vi "Sort Classes by Name.vi"(8 "error in (no error)":errorcluster, 11 "Classes":refnum<vi>[](array[refnum])) -> (0 "error out":errorcluster, 3 "Sorted Classes":refnum<vi>[](array[refnum]))   [LabVIEW 2020, in "Peek Window.lvlib" / "Dynamic Dispatch VI Type.lvclass"]
uses:
  Dynamic Dispatch VI Type.lvclass
  Dynamic Dispatch VI Type.lvclass/Dynamic Dispatch VI Type.ctl
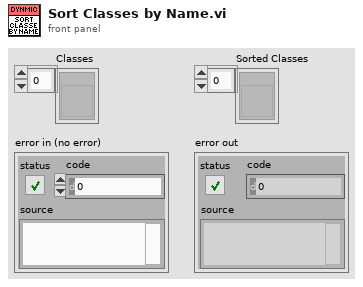
[diagram p1: front panel]
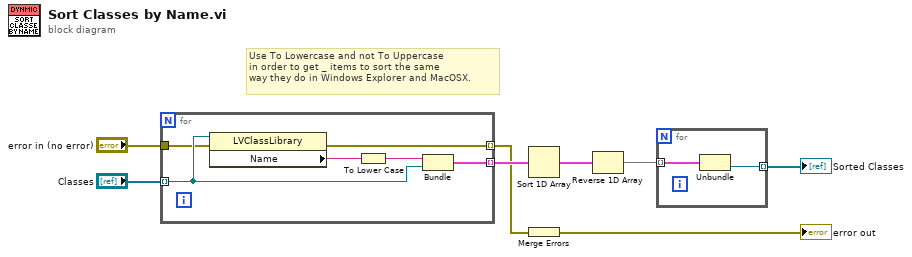
[diagram p0: block diagram]
diagram:
  # "Use To Lowercase and not To Uppercase\nin order to get _ items to sort the same\nway they do in Windows Explorer and MacOSX."
  n1 = for {
    tunnel: "Classes" -> [w13] mode=indexing
    tunnel: [w12] -> w4 mode=indexing
    tunnel: "error in (no error)" -> [w10]
    tunnel: [w9] -> w2 mode=indexing
    n2 = property class="LVClassLibrary"(reference=w13, error in=w10) -> (error out=w9:errorcluster, "Name"=w14:string)  [unwired: 1 out]
    n3 = To Lower Case(string=w14) -> (all lower case string=w11:string)
    n4 = Bundle(w11, w13) -> (w12:cluster{string, refnum<vi>})  [unwired: 1 in]
  }
  n5 = Sort 1D Array(array=w4) -> (sorted array=w5:cluster{string, refnum<vi>}[])
  n6 = Merge Errors(w2) -> (→"error out":errorcluster)
  n7 = Reverse 1D Array(array=w5) -> (reversed array=w8:cluster{string, refnum<vi>}[])
  n8 = for {
    tunnel: w8 -> [w16] mode=indexing
    tunnel: [w15] -> w7 mode=indexing
    n9 = Unbundle(w16) -> (w15:refnum<vi>)  [unwired: 1 out]
  }
  "Sorted Classes" <- w7
